vi "write_y.vi"(8 "error in (no error)":errorcluster, 10 "y":dbl[](array[numeric]), 11 "LogisticRegressionCV in":refnum<class "LogisticRegressionCV.lvclass">) -> (0 "error out":errorcluster, 3 "LogisticRegressionCV out":refnum<class "LogisticRegressionCV.lvclass">)   [LabVIEW 2020, in "LogisticRegressionCV.lvclass"]
uses:
  LogisticRegressionCV.lvclass
  LogisticRegressionCV.lvclass/LogisticRegressionCV.ctl
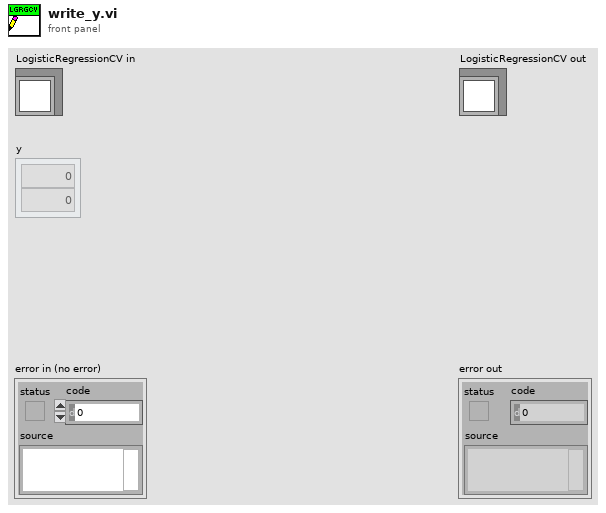
[diagram p1: front panel]
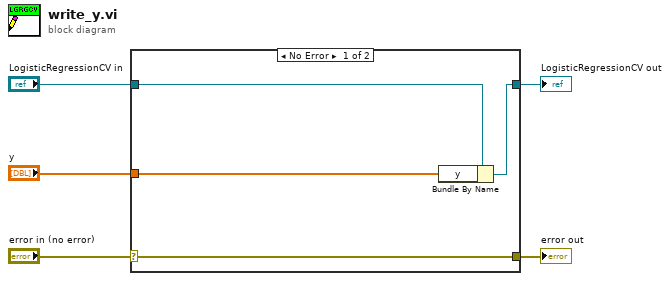
[diagram p0: block diagram]
diagram:
  n1 = case shown="No Error" "error in (no error)" {
    selector: "error in (no error)" -> [w9 w10]
    tunnel: [w9 w10] -> w4
    tunnel: [w7 w11] -> w2
    tunnel: "LogisticRegressionCV in" -> [w8 w11]
    tunnel: "y" -> [w6 _]
    frame No Error {
      n2 = Bundle By Name(cluster=w8, "y"=w6) -> (w7:refnum<class "LogisticRegressionCV.lvclass">)
    }
    frame Error {
    }
  }
  "error out" <- w4
  "LogisticRegressionCV out" <- w2
